vi "Convert Error Cluster to Table.vi"(11 "Error Codes":cluster{i32, string}[](array[cluster])) -> (2 "Code":i32[](array[numeric]), 3 "String":string[](array[string]))   [LabVIEW 2019, in "Protection and Counter Addon System Explorer.lvlib"] (continued)
(Hex 0xFFFFFCB6) The timed structure failed to unreserve the NI Scan Engine."}, {-841, "LabVIEW: (Hex 0xFFFFFCB7) The timed structure failed to retrieve the NI Scan Engine mode."}, {-840, "LabVIEW: (Hex 0xFFFFFCB8) The timed structure failed to reserve the NI Scan Engine."}, {-832, "LabVIEW: (Hex 0xFFFFFCC0) The Priority Mapper Table is full."}, {-831, "LabVIEW: (Hex 0xFFFFFCC1) Timing Source Fire Count Overflow"}, {-830, "LabVIEW: (Hex 0xFFFFFCC2) Invalid Trigger ID"}, {-826, "LabVIEW: (Hex 0xFFFFFCC6) A time-critical VI contains a timed structure."}, {-825, "LabVIEW: (Hex 0xFFFFFCC7) Invalid CPU Specified for timed structure."}, {-823, "LabVIEW: (Hex 0xFFFFFCC9) Cannot load Timed Loop Scheduler Dynamic Library."}, {-822, "LabVIEW: (Hex 0xFFFFFCCA) The timed structure feature or type is not supported on the current platform for the following timing source."}, {-821, "LabVIEW: (Hex 0xFFFFFCCB) The following timed structures timed out while waiting for the synchronization group to synchronize all timed structures in the group."}, {-820, "LabVIEW: (Hex 0xFFFFFCCC) The following timed structure has been initialized with illegal parameters."}, {-819, "LabVIEW: (Hex 0xFFFFFCCD) An illegal mode has been specified for the following given Timed Loop."}, {-818, "LabVIEW: (Hex 0xFFFFFCCE) An illegal period, priority, deadline, offset, or start has been specified for the following timed structure."}, {-817, "LabVIEW: (Hex 0xFFFFFCCF) Timing Source error or attempted to execute another iteration of a Timed Loop that was already aborted due to an error of the following timing source."}, {-816, "LabVIEW: (Hex 0xFFFFFCD0) Timed structure aborted or attempted to execute another iteration of the following aborted Timed Loop."}, {-815, "LabVIEW: (Hex 0xFFFFFCD1) Cannot add timing source to the following active timing source hierarchy."}, {-814, "LabVIEW: (Hex 0xFFFFFCD2) Cannot add timed structure to the active timed structure synchronization group."}, {-813, "LabVIEW: (Hex 0xFFFFFCD3) The following timing source can be assigned to only one timing source hierarchy at a time."}, {-812, "LabVIEW: (Hex 0xFFFFFCD4) The following timed structure can only be assigned to one timed structure synchronization group at a time."}, {-811, "LabVIEW: (Hex 0xFFFFFCD5) The given name is already being used by another timing source hierarchy:"}, {-810, "LabVIEW: (Hex 0xFFFFFCD6) The given name is already being used by another timed structure synchronization group:"}, {-809, "LabVIEW: (Hex 0xFFFFFCD7) The given name is already being used by the following timing source."}, {-808, "LabVIEW: (Hex 0xFFFFFCD8) The given name is already being used by the following timed structure."}, {-807, "LabVIEW: (Hex 0xFFFFFCD9) The following timing source hierarchy does not exist possibly because the timing source hierarchy has never been created, has been cleared, or an illegal action was attempted."}, {-806, "LabVIEW: (Hex 0xFFFFFCDA) The following synchronization group does not exist possibly because the synchronization group has never been created, has been cleared, or an illegal action was attempted."}, {-805, "LabVIEW: (Hex 0xFFFFFCDB) The following timing source does not exist. This error might occur because the timing source was never created, has been cleared, or an illegal action was attempted. Use the Create Timing Source VI to create a Timed Loop timing source."}, {-804, "LabVIEW: (Hex 0xFFFFFCDC) The timed structure does not exist, possibly because the timed structure has not been created, the timed structure has been cleared, or an illegal operation was attempted."}, {-803, "LabVIEW: (Hex 0xFFFFFCDD) Creating a new timing source hierarchy exceeds the maximum allowed number of simultaneously active timing source hierarchies."}, {-802, "LabVIEW: (Hex 0xFFFFFCDE) Creating another timed structure synchronization group exceeds the maximum allowed number of simultaneously active synchronization groups."}, {-801, "LabVIEW: (Hex 0xFFFFFCDF) Creating another timing source exceeds the maximum allowed number of simultaneously active timing sources."}, {-800, "LabVIEW: (Hex 0xFFFFFCE0) Creating another timed structure exceeds the maximum allowed number of simultaneously active timed structures."}, {-722, "LabVIEW: (Hex 0xFFFFFD2E) The TEDS bitstream is invalid or corrupt."}, {-721, "LabVIEW: (Hex 0xFFFFFD2F) The specified index is outside the bounds of the TEDS data array."}, {-720, "LabVIEW: (Hex 0xFFFFFD30) The specified value is outside of the acceptable range for this property."}, {-719, "LabVIEW: (Hex 0xFFFFFD31) The Basic TEDS was not found in the TEDS data."}, {-718, "LabVIEW: (Hex 0xFFFFFD32) LabVIEW is unable to locate the specified SelectCase or StructArray."}, {-717, "LabVIEW: (Hex 0xFFFFFD33) The specified VTEDS file was written with an incompatible version of the TEDS library."}, {-716, "LabVIEW: (Hex 0xFFFFFD34) The EEPROM is too small for data."}, {-715, "LabVIEW: (Hex 0xFFFFFD35) EEPROM Write Failure"}, {-714, "LabVIEW: (Hex 0xFFFFFD36) Bad EEPROM ID"}, {-713, "LabVIEW: (Hex 0xFFFFFD37) No EEPROM is detected."}, {-712, "LabVIEW: (Hex 0xFFFFFD38) This property cannot be edited because it is a constant in the template for this sensor."}, {-711, "LabVIEW: (Hex 0xFFFFFD39) The enumeration for this property does not correspond to the data type specified by the template."}, {-710, "LabVIEW: (Hex 0xFFFFFD3A) This TEDS sensor requires a manufacturer defined template."}, {-709, "LabVIEW: (Hex 0xFFFFFD3B) The specified property is a floating-point data type according to the template. Casting this property to an unsigned integer will result in a loss of precision."}, {-708, "LabVIEW: (Hex 0xFFFFFD3C) The specified property is specified by the TEDS template as a string data type and cannot be converted to a numeric."}, {-707, "LabVIEW: (Hex 0xFFFFFD3D) The TEDS user data does not contain 7-bit ASCII code."}, {-706, "LabVIEW: (Hex 0xFFFFFD3E) The requested property cannot be found in the current TEDS data."}, {-705, "LabVIEW: (Hex 0xFFFFFD3F) The template to decode the remainder of the TEDS bitstream cannot be found in the specified template directory."}, {-704, "LabVIEW: (Hex 0xFFFFFD40) The header selector in the legacy Basic TEDS is outside the acceptable range."}, {-703, "LabVIEW: (Hex 0xFFFFFD41) The TEDS data checksum is invalid."}, {-702, "LabVIEW: (Hex 0xFFFFFD42) This VI does not support the data type for this property."}, {-701, "LabVIEW: (Hex 0xFFFFFD43) The number of bits required for the requested action is not divisible by five."}, {-700, "LabVIEW: (Hex 0xFFFFFD44) The number of bits required is not divisible by seven."}, {-620, "LabVIEW: (Hex 0xFFFFFD94) Networked machine was not found."}, {-619, "LabVIEW: (Hex 0xFFFFFD95) Remote registry services not available or remote administration not enabled."}, {-618, "LabVIEW: (Hex 0xFFFFFD96) Cannot create a stable subkey under a volatile parent key."}, {-617, "LabVIEW: (Hex 0xFFFFFD97) Cannot create a symbolic link in a registry key that already has subkeys or values."}, {-616, "LabVIEW: (Hex 0xFFFFFD98) System could not allocate the required space in a registry log."}, {-615, "LabVIEW: (Hex 0xFFFFFD99) Illegal operation attempted on a registry key that has been marked for deletion."}, {-614, "LabVIEW: (Hex 0xFFFFFD9A) The system has attempted to load or restore a file into the registry, but the specified file is not in a registry file format."}, {-613, "LabVIEW: (Hex 0xFFFFFD9B) An I/O operation initiated by the registry failed irrecoverably. The registry could not read in, or write out, or flush, one of the files that contain the system's image of the registry."}, {-612, "LabVIEW: (Hex 0xFFFFFD9C) The registry is corrupted. The structure of one of the files that contains registry data is corrupted, the system's image of the file in memory is corrupted, or the file could not be recovered because the alternate copy or log was absent or corrupted."}, {-611, "LabVIEW: (Hex 0xFFFFFD9D) One of the files in the registry database had to be recovered by use of a log or alternate copy. The recovery was successful."}, {-610, "LabVIEW: (Hex 0xFFFFFD9E) The configuration registry key could not be written."}, {-609, "LabVIEW: (Hex 0xFFFFFD9F) The configuration registry key could not be read."}, {-608, "LabVIEW: (Hex 0xFFFFFDA0) The configuration registry key could not be opened."}, {-607, "LabVIEW: (Hex 0xFFFFFDA1) The configuration registry key is invalid."}, {-606, "LabVIEW: (Hex 0xFFFFFDA2) The configuration registry database is corrupt."}, {-605, "LabVIEW: (Hex 0xFFFFFDA3) Attempted to read beyond last key or value."}, {-604, "LabVIEW: (Hex 0xFFFFFDA4) Remote registry access denied."}, {-603, "LabVIEW: (Hex 0xFFFFFDA5) Specified key or value does not exist."}, {-602, "LabVIEW: (Hex 0xFFFFFDA6) Invalid registry refnum."}, {-601, "LabVIEW: (Hex 0xFFFFFDA7) Incorrect data type specified."}, {-600, "LabVIEW: (Hex 0xFFFFFDA8) Undetermined Windows registry error."}, {0, "LabVIEW: (Hex 0x0) Error connecting to GPIB driver or device. The NI-488.2 driver may not be installed."}, {1, "LabVIEW: (Hex 0x1) An input parameter is invalid. For example if the input is a path, the path might contain a character not allowed by the OS such as ? or @."}, {2, "LabVIEW: (Hex 0x2) Memory is full."}, {3, "LabVIEW: (Hex 0x3) Internal error. Wrong memory zone accessed."}, {4, "LabVIEW: (Hex 0x4) End of file encountered."}, {5, "LabVIEW: (Hex 0x5) File already open."}, {6, "LabVIEW: (Hex 0x6) Generic file I/O error."}, {7, "LabVIEW: (Hex 0x7) File not found. The file might be in a different location or deleted. Use the command prompt or the file explorer to verify that the path is correct."}, {8, "LabVIEW: (Hex 0x8) File permission error. You do not have the correct permissions for the file."}, {9, "LabVIEW: (Hex 0x9) Disk full. The disk or hard drive does not have enough free space to complete the operation. Try freeing up disk space or saving to a different disk or drive."}, {10, "LabVIEW: (Hex 0xA) Duplicate path."}, {11, "LabVIEW: (Hex 0xB) Too many files open."}, {12, "LabVIEW: (Hex 0xC) Some system capacity necessary for operation is not enabled."}, {13, "LabVIEW: (Hex 0xD) Failed to load dynamic library because of missing external symbols or dependencies, or because of an invalid file format."}, {14, "LabVIEW: (Hex 0xE) Cannot add resource."}, {15, "LabVIEW: (Hex 0xF) Resource not found."}, {16, "LabVIEW: (Hex 0x10) Image not found."}, {17, "LabVIEW: (Hex 0x11) Not enough memory to manipulate image."}, {18, "LabVIEW: (Hex 0x12) Pen does not exist."}, {19, "LabVIEW: (Hex 0x13) Configuration type invalid."}, {20, "LabVIEW: (Hex 0x14) Configuration token not found."}, {21, "LabVIEW: (Hex 0x15) Error occurred parsing configuration string."}, {22, "LabVIEW: (Hex 0x16) Configuration memory error."}, {23, "LabVIEW: (Hex 0x17) Bad external code format."}, {24, "LabVIEW: (Hex 0x18) External subroutine not supported."}, {25, "LabVIEW: (Hex 0x19) External code not present."}, {26, "LabVIEW: (Hex 0x1A) Null window."}, {27, "LabVIEW: (Hex 0x1B) Destroy window error."}, {28, "LabVIEW: (Hex 0x1C) Null menu."}, {29, "LabVIEW: (Hex 0x1D) Print aborted."}, {30, "LabVIEW: (Hex 0x1E) Bad print record."}, {31, "LabVIEW: (Hex 0x1F) Print driver error."}, {32, "LabVIEW: (Hex 0x20) Operating system error during print."}, {33, "LabVIEW: (Hex 0x21) Memory error during print."}, {34, "LabVIEW: (Hex 0x22) Print dialog error."}, {35, "LabVIEW: (Hex 0x23) Generic print error."}, {36, "LabVIEW: (Hex 0x24) Invalid device refnum."}, {37, "LabVIEW: (Hex 0x25) Device not found."}, {38, "LabVIEW: (Hex 0x26) Device parameter error."}, {39, "LabVIEW: (Hex 0x27) Device unit error."}, {40, "LabVIEW: (Hex 0x28) Cannot open device."}, {41, "LabVIEW: (Hex 0x29) Device call aborted."}, {42, "LabVIEW: (Hex 0x2A) Generic error."}, {43, "LabVIEW: (Hex 0x2B) Operation cancelled by user."}, {44, "LabVIEW: (Hex 0x2C) Object ID too low."}, {45, "LabVIEW: (Hex 0x2D) Object ID too high."}, {46, "LabVIEW: (Hex 0x2E) Object not in heap."}, {47, "LabVIEW: (Hex 0x2F) Unknown heap."}, {48, "LabVIEW: (Hex 0x30) Unknown object (invalid DefProc)."}, {49, "LabVIEW: (Hex 0x31) Unknown object (DefProc not in table)."}, {50, "LabVIEW: (Hex 0x32) Message out of range."}, {51, "LabVIEW: (Hex 0x33) Null method."}, {52, "LabVIEW: (Hex 0x34) Unknown message."}, {53, "LabVIEW: (Hex 0x35) Manager call not supported."}, {54, "LabVIEW: (Hex 0x36) The network address is ill-formed. Make sure the address is in a valid format. For TCP/IP, the address can be either a machine name or an IP address in the form xxx.xxx.xxx.xxx. If this error occurs when specifying a machine name, make sure the machine name is valid. Try to ping the machine name. Check that you have a DNS server properly configured. If you are using the TCP Open Connection function, ensure that the value of the remote port or service name is not 0."}, {55, "LabVIEW: (Hex 0x37) The network operation is in progress."}, {56, "LabVIEW: (Hex 0x38) The network operation exceeded the user-specified or system time limit."}, {57, "LabVIEW: (Hex 0x39) The network connection is busy."}, {58, "LabVIEW: (Hex 0x3A) The network function is not supported by the system."}, {59, "LabVIEW: (Hex 0x3B) The network is down, unreachable, or has been reset."}, {60, "LabVIEW: (Hex 0x3C) The specified port or network address is currently in use. Select an available port or network address."}, {61, "LabVIEW: (Hex 0x3D) Serial port parity error."}, {61, "LabVIEW: (Hex 0x3D) The system could not allocate the necessary memory."}, {62, "LabVIEW: (Hex 0x3E) Serial port overrun error."}, {62, "LabVIEW: (Hex 0x3E) The system caused the network connection to be aborted."}, {63, "LabVIEW: (Hex 0x3F) Serial port receive buffer overflow."}, {63, "LabVIEW: (Hex 0x3F) The network connection was refused by the server."}, {64, "LabVIEW: (Hex 0x40) Serial port framing error."}, {64, "LabVIEW: (Hex 0x40) The network connection is not yet established."}, {65, "LabVIEW: (Hex 0x41) Serial port timeout; bytes not received at serial port."}, {65, "LabVIEW: (Hex 0x41) The network connection is already established."}, {66, "LabVIEW: (Hex 0x42) The network connection was closed by the peer. If you are using the Open VI Reference function on a remote VI Server connection, verify that the machine is allowed access by selecting <b>Tools>>Options>>VI Server</b> on the server side."}, {67, "LabVIEW: (Hex 0x43) Interapplication Manager initialization error."}, {68, "LabVIEW: (Hex 0x44) Bad occurrence."}, {69, "LabVIEW: (Hex 0x45) Handler does not know what occurrence to wait for."}, {70, "LabVIEW: (Hex 0x46) Occurrence queue overflow."}, {71, "LabVIEW: (Hex 0x47) File datalog type conflict."}, {72, "LabVIEW: (Hex 0x48) Semaphore not signaled."}, {73, "LabVIEW: (Hex 0x49) Interapplication Manager unrecognized type error."}, {74, "LabVIEW: (Hex 0x4A) Memory or data structure corrupt."}, {75, "LabVIEW: (Hex 0x4B) Failed to make temporary DLL."}, {76, "LabVIEW: (Hex 0x4C) Old CIN version."}, {81, "LabVIEW: (Hex 0x51) Format specifier type mismatch."}, {82, "LabVIEW: (Hex 0x52) Unknown format specifier."}, {83, "LabVIEW: (Hex 0x53) Too few format specifiers."}, {84, "LabVIEW: (Hex 0x54) Too many format specifiers."}, {85, "LabVIEW: (Hex 0x55) Scan failed. The input string does not contain data in the expected format."}, {87, "LabVIEW: (Hex 0x57) Error converting to variant."}, {88, "LabVIEW: (Hex 0x58) Run-time menu error."}, {89, "LabVIEW: (Hex 0x59) Another user tampered with the VI password."}, {90, "LabVIEW: (Hex 0x5A) Variant attribute not found."}, {91, "LabVIEW: (Hex 0x5B) The data type of the variant is not compatible with the data type wired to the type input."}, {92, "LabVIEW: (Hex 0x5C) The ActiveX event data was not available on the queue."}, {93, "LabVIEW: (Hex 0x5D) ActiveX event information was not available."}, {94, "LabVIEW: (Hex 0x5E) The occurrence associated with the ActiveX event was not found."}, {95, "LabVIEW: (Hex 0x5F) The ActiveX event queue could not be created."}, {96, "LabVIEW: (Hex 0x60) ActiveX event information was not available in the type library."}, {97, "LabVIEW: (Hex 0x61) A null or previously deleted refnum was passed in as an input."}, {98, "LabVIEW: (Hex 0x62) Incorrect file type. Attempted to read from or write to a file of a type incompatible with the operation. This normally is a user data file."}, {99, "LabVIEW: (Hex 0x63) Incorrect file version. Attempted to read from or write to a file of a version incompatible with the write/read function version. This file normally is a user data file."}, {100, "LabVIEW: (Hex 0x64) File contains erroneous data. This normally is a user data file."}, {102, "LabVIEW: (Hex 0x66) IVI invalid downcast."}, {103, "LabVIEW: (Hex 0x67) No IVI class session opened.  You must call the class driver Initialize VI before you can call a specific driver VI.  This error also can occur if the IVI Logical Name control is set to the wrong IVI Class."}, {108, "LabVIEW: (Hex 0x6C) Singlecast connections cannot send to multicast addresses."}, {109, "LabVIEW: (Hex 0x6D) Multicast connections cannot send to singlecast addresses."}, {110, "LabVIEW: (Hex 0x6E) Specified IP address is not in multicast address range."}, {111, "LabVIEW: (Hex 0x6F) Cannot write to read-only multicast connection."}, {112, "LabVIEW: (Hex 0x70) Cannot read from write-only multicast connection."}, {113, "LabVIEW: (Hex 0x71) A message sent on a datagram socket was larger than the internal message buffer or some other network limit, or the buffer used to receive a datagram was smaller than the datagram itself."}, {114, "LabVIEW: (Hex 0x72) Could not create TCP listener port because the port, service name, or net address conflict with a TCP listener that already exists."}, {116, "LabVIEW: (Hex 0x74) Unflatten or byte stream read operation failed due to corrupt, unexpected, or truncated data."}, {117, "LabVIEW: (Hex 0x75) Directory path supplied where a file path is required."}, {118, "LabVIEW: (Hex 0x76) The supplied folder path does not exist."}, {119, "LabVIEW: (Hex 0x77) Illegal combination of Bluetooth discoverable and non-connectable modes."}, {120, "LabVIEW: (Hex 0x78) Error setting Bluetooth mode."}, {121, "LabVIEW: (Hex 0x79) Invalid GUID string."}, {122, "LabVIEW: (Hex 0x7A) The resource you are attempting to open was created in a more recent version of LabVIEW and is incompatible with this version."}, {123, "LabVIEW: (Hex 0x7B) A timeout occurred."}, {124, "LabVIEW: (Hex 0x7C) A string contained an unexpected null character."}, {125, "LabVIEW: (Hex 0x7D) A stack overflow occurred."}, {126, "LabVIEW: (Hex 0x7E) Could not query socket state."}, {127, "LabVIEW: (Hex 0x7F) The specified socket is not an IPv4 socket."}, {128, "LabVIEW: (Hex 0x80) Open connection limit exceeded."}, {129, "LabVIEW: (Hex 0x81) The path to access is too long for the current operating system."}, {130, "LabVIEW: (Hex 0x82) Operation attempted to create a set with duplicate elements. All elements of a set must be unique."}, {131, "LabVIEW: (Hex 0x83) Operation attempted to create a map with duplicate keys. All keys of a map must be unique."}, {824, "LabVIEW: (Hex 0x338) You must  supply a mode to change the offset of the Timed Loop."}, {1000, "LabVIEW: (Hex 0x3E8) The VI is not in a state compatible with this operation."}, {1001, "LabVIEW: (Hex 0x3E9) The VI front panel is not open."}, {1002, "LabVIEW: (Hex 0x3EA) The VI cannot run because it has a front panel control in an error state."}, {1003, "LabVIEW: (Hex 0x3EB) The VI is not executable.  This error may occur because the VI is either broken or contains a subVI that LabVIEW cannot locate. Select <b>File>>Open</b> to open the VI and verify that you can run it."}, {1004, "LabVIEW: (Hex 0x3EC) The VI is not in memory."}, {1005, "LabVIEW: (Hex 0x3ED) VI execution has been disabled in the <b>VI Properties</b> dialog box."}, {1006, "LabVIEW: (Hex 0x3EE) FPDCO on connector pane thinks it is constant."}, {1007, "LabVIEW: (Hex 0x3EF) No IP record in summary."}, {1008, "LabVIEW: (Hex 0x3F0) Cannot load connector pane."}, {1009, "LabVIEW: (Hex 0x3F1) Variant tag out of range."}, {1010, "LabVIEW: (Hex 0x3F2) No default or operate data."}, {1011, "LabVIEW: (Hex 0x3F3) VI Creation failed."}, {1012, "LabVIEW: (Hex 0x3F4) Cannot load block diagram."}, {1013, "LabVIEW: (Hex 0x3F5) Cannot load front panel."}, {1014, "LabVIEW: (Hex 0x3F6) Linker error."}, {1015, "LabVIEW: (Hex 0x3F7) Printer is not responding. Check printer configuration."}, {1016, "LabVIEW: (Hex 0x3F8) Cannot load History."}, {1017, "LabVIEW: (Hex 0x3F9) VI has been modified on disk since it was last loaded or saved."}, {1018, "LabVIEW: (Hex 0x3FA) Unspecified error occurred."}, {1019, "LabVIEW: (Hex 0x3FB) One or more untitled subVIs exist. This file cannot be saved until all dependent files have been named."}, {1020, "LabVIEW: (Hex 0x3FC) This CIN can only be invoked from a registered wizard."}, {1021, "LabVIEW: (Hex 0x3FD) Illegal Object Id passed to wizard CIN."}, {1022, "LabVIEW: (Hex 0x3FE) Wizard Template not found."}, {1023, "LabVIEW: (Hex 0x3FF) Wizard template does not have a diagram."}, {1024, "LabVIEW: (Hex 0x400) Call Instrument aborted."}, {1025, "LabVIEW: (Hex 0x401) Application Reference is invalid."}, {1026, "LabVIEW: (Hex 0x402) VI Reference is invalid."}, {1027, "LabVIEW: (Hex 0x403) For the requested operation, the reference cannot be reserved as requested, is in an improper reservation mode, or the execution state must be set to running or reserved."}, {1028, "LabVIEW: (Hex 0x404) Attribute selector is invalid."}, {1029, "LabVIEW: (Hex 0x405) VI Server property is read-only."}, {1030, "LabVIEW: (Hex 0x406) VI Reference is already reserved for editing."}, {1031, "LabVIEW: (Hex 0x407) VI Reference type does not match VI connector pane."}, {1032, "LabVIEW: (Hex 0x408) VI Server access denied."}, {1033, "LabVIEW: (Hex 0x409) Bad run-time menu file version."}, {1034, "LabVIEW: (Hex 0x40A) Bad run-time menu file."}, {1035, "LabVIEW: (Hex 0x40B) Operation is invalid for this type of VI."}, {1036, "LabVIEW: (Hex 0x40C) Method selector is invalid."}, {1037, "LabVIEW: (Hex 0x40D) Incompatible VI Server protocol version."}, {1038, "LabVIEW: (Hex 0x40E) Required parameter missing."}, {1039, "LabVIEW: (Hex 0x40F) VI was aborted."}, {1040, "LabVIEW: (Hex 0x410) VI is password protected."}, {1041, "LabVIEW: (Hex 0x411) Incorrect password."}, {1042, "LabVIEW: (Hex 0x412) Attempted recursive call."}, {1043, "LabVIEW: (Hex 0x413) The property or method is not supported in this version of LabVIEW."}, {1044, "LabVIEW: (Hex 0x414) VI is locked."}, {1045, "LabVIEW: (Hex 0x415) Null Refnum passed to Close Reference."}, {1046, "LabVIEW: (Hex 0x416) LabVIEW cannot initialize the script server.  Ensure the server software is installed."}, {1047, "LabVIEW: (Hex 0x417) LabVIEW failed to send variable to the script server."}, {1048, "LabVIEW: (Hex 0x418) LabVIEW failed to get variable from the script server."}, {1049, "LabVIEW: (Hex 0x419) LabVIEW failed to send script text to the script server."}, {1050, "LabVIEW: (Hex 0x41A) Error occurred while executing script."}, {1051, "LabVIEW: (Hex 0x41B) A LabVIEW file of that name already exists in memory, or exists within a project library already in memory."}, {1052, "LabVIEW: (Hex 0x41C) The LabVIEW filename is invalid."}, {1053, "LabVIEW: (Hex 0x41D) At run time, LabVIEW cannot find script support DLL."}, {1054, "LabVIEW: (Hex 0x41E) The specified object was not found."}, {1055, "LabVIEW: (Hex 0x41F) Object reference is invalid."}, {1056, "LabVIEW: (Hex 0x420) Specified object is not scriptable in this version."}, {1057, "LabVIEW: (Hex 0x421) Type mismatch: Object cannot be cast to the specified type."}, {1058, "LabVIEW: (Hex 0x422) Specified property not found."}, {1059, "LabVIEW: (Hex 0x423) Unexpected file type."}, {1060, "LabVIEW: (Hex 0x424) Object cannot contain (own) the specified object."}, {1061, "LabVIEW: (Hex 0x425) Unable to create new object."}, {1062, "LabVIEW: (Hex 0x426) Specified objects cannot be wired together."}, {1063, "LabVIEW: (Hex 0x427) Specified terminal not found in the object."}, {1064, "LabVIEW: (Hex 0x428) The specified VI may not be saved for previous because it resides in the vi.lib directory."}, {1065, "LabVIEW: (Hex 0x429) The path to the VI to save is an empty or relative path.  It must be an absolute path."}, {1066, "LabVIEW: (Hex 0x42A) Hardware open error."}, {1067, "LabVIEW: (Hex 0x42B) Hardware close error."}, {1068, "LabVIEW: (Hex 0x42C) Hardware transact error."}, {1069, "LabVIEW: (Hex 0x42D) Hardware DLL missing."}, {1070, "LabVIEW: (Hex 0x42E) Hardware no session error."}, {1071, "LabVIEW: (Hex 0x42F) LabVIEW cannot locate the specified method."}, {1072, "LabVIEW: (Hex 0x430) This property or method is not yet implemented."}, {1073, "LabVIEW: (Hex 0x431) This property is writable only when the VI is in edit mode, or this method is available only when the VI is in edit mode."}, {1074, "LabVIEW: (Hex 0x432) Cannot create a control/indicator for the specified terminal."}, {1075, "LabVIEW: (Hex 0x433) Cannot create a constant for the specified terminal."}, {1076, "LabVIEW: (Hex 0x434) VI is not debuggable."}, {1077, "LabVIEW: (Hex 0x435) Invalid property value."}, {1078, "LabVIEW: (Hex 0x436) Failed to load shared library %s. Ensure that the library is present on the RT target. Use either MAX to install NI software or FTP to transfer custom libraries to the RT target."}, {1079, "LabVIEW: (Hex 0x437) When the RT target booted, the startup application configured to launch was missing."}, {1080, "LabVIEW: (Hex 0x438) The startup application configured to launch was corrupt and failed to load when the RT target booted."}, {1081, "LabVIEW: (Hex 0x439) Exception caused by loading of library %s on RT target device."}, {1082, "LabVIEW: (Hex 0x43A) Operation not valid for strict type definition instance."}, {1083, "LabVIEW: (Hex 0x43B) Invalid connector pane pattern."}, {1084, "LabVIEW: (Hex 0x43C) Specified control or indicator cannot be hooked up to the connector pane."}, {1085, "LabVIEW: (Hex 0x43D) Invalid connector terminal."}, {1086, "LabVIEW: (Hex 0x43E) Wrong control type."}, {1087, "LabVIEW: (Hex 0x43F) There is no DataSocket information available for the object."}, {1088, "LabVIEW: (Hex 0x440) Bad value for parameter."}, {1089, "LabVIEW: (Hex 0x441) Error occurred while executing script. Error message from server: %s."}, {1090, "LabVIEW: (Hex 0x442) Specified object cannot be moved."}, {1091, "LabVIEW: (Hex 0x443) The VI Server or client received an unrecognized message."}, {1092, "LabVIEW: (Hex 0x444) Invalid Class Operator VI."}, {1093, "LabVIEW: (Hex 0x445) Specified object is not deletable."}, {1094, "LabVIEW: (Hex 0x446) Queue and notifier references of the same name must be obtained using the same data type."}, {1095, "LabVIEW: (Hex 0x447) This container cannot be left without a subtype. Right-click the container border and select Replace or drag new subtype."}, {1096, "LabVIEW: (Hex 0x448) The Open VI Reference function cannot prepare a non-reentrant VI for reentrant run."}, {1097, "LabVIEW: (Hex 0x449) An exception occurred within the external code called by a Call Library Function Node. The exception might have corrupted the LabVIEW memory. Save any work to a new location and restart LabVIEW."}, {1098, "LabVIEW: (Hex 0x44A) Cannot disconnect type definitions or polymorphic VIs if the block diagram is not available."}, {1099, "LabVIEW: (Hex 0x44B) Scripting: SubVI is not loaded."}, {1100, "LabVIEW: (Hex 0x44C) No object of that name was found. No reference could be returned."}, {1101, "LabVIEW: (Hex 0x44D) Insufficient privileges to read, write, or create an item in the DataSocket Server. Use the DataSocket Server Manager to configure these privileges."}, {1102, "LabVIEW: (Hex 0x44E) The string wired to the <b>xml string</b> input is empty."}, {1103, "LabVIEW: (Hex 0x44F) The XML tag describing the type of data is not recognized."}, {1104, "LabVIEW: (Hex 0x450) No end tag was found for an XML start/end tag pair."}, {1105, "LabVIEW: (Hex 0x451) An unknown or unexpected XML tag was discovered."}, {1106, "LabVIEW: (Hex 0x452) The XML tag describing the type of data does not match the wired type."}, {1107, "LabVIEW: (Hex 0x453) The XML enumerated type choice(s) does not match the wired type."}, {1108, "LabVIEW: (Hex 0x454) XML value text is illegal or out of range for type and/or format."}, {1109, "LabVIEW: (Hex 0x455) Unsupported data type."}, {1110, "LabVIEW: (Hex 0x456) No longer used."}, {1111, "LabVIEW: (Hex 0x457) Release Semaphore called on a semaphore that was not currently acquired."}, {1112, "LabVIEW: (Hex 0x458) Internal Error. No class manager found for the type requested."}, {1113, "LabVIEW: (Hex 0x459) Internal Error. The external object class was not found."}, {1114, "LabVIEW: (Hex 0x45A) This item is read-only. You must connect in read mode."}, {1115, "LabVIEW: (Hex 0x45B) This item is write-only. You must connect in write mode."}, {1116, "LabVIEW: (Hex 0x45C) RTTarget.DiskCache.SizeInKB config token must be greater than zero."}, {1117, "LabVIEW: (Hex 0x45D) RTTarget.DiskCache.Thread.Priority config token must be between -2 and 2."}, {1118, "LabVIEW: (Hex 0x45E) RTTarget.DiskCache.Thread.IntervalInSecs config token must be greater than zero."}, {1119, "LabVIEW: (Hex 0x45F) RTTarget.DiskCache.Thread.LinePerWakeup config token must be greater than or equal to zero."}, {1120, "LabVIEW: (Hex 0x460) Not enough memory to create disk cache."}, {1121, "LabVIEW: (Hex 0x461) Cannot create disk cache flush thread."}, {1122, "LabVIEW: (Hex 0x462) Refnum became invalid while node waited for it."}, {1123, "LabVIEW: (Hex 0x463) You cannot create an object (such as control caption) in built applications. You must create these objects in the LabVIEW development system."}, {1124, "LabVIEW: (Hex 0x464) VI is not loadable.\n\nIn a built application, this error might occur because the VI being loaded was last compiled for a different OS or with CPU features, such as SSE, that this target does not support. In this case you must rebuild the application for the target OS and make sure SSE compiler settings in the build specifications match the target platform. This error also might occur if the VI is a polymorphic VI, which cannot be loaded in the LabVIEW Run-Time Engine. You must load an instance of the polymorphic VI instead of the polymorphic VI itself."}, {1125, "LabVIEW: (Hex 0x465) File version is later than the current LabVIEW version."}, {1126, "LabVIEW: (Hex 0x466) VI version is too early to convert to the current LabVIEW version."}, {1127, "LabVIEW: (Hex 0x467) Cannot instantiate template VI because it is already in memory."}, {1128, "LabVIEW: (Hex 0x468) Input unit is not compatible with the current unit."}, {1129, "LabVIEW: (Hex 0x469) You cannot assign the same numeric value to two or more strings in a ring control. You also cannot assign the same string value to two or more strings in a combo box control."}, {1130, "LabVIEW: (Hex 0x46A) The VI Server connection peer is unresponsive. Refer to the Connection Responsiveness: Check Method topic in the LabVIEW Help for more information about connection polling."}, {1131, "LabVIEW: (Hex 0x46B) You cannot use this property with this system control."}, {1132, "LabVIEW: (Hex 0x46C) Busy with another operation."}, {1133, "LabVIEW: (Hex 0x46D) LabVIEW is busy connecting."}, {1134, "LabVIEW: (Hex 0x46E) A different read operation is in progress."}, {1135, "LabVIEW: (Hex 0x46F) The tree control's active item is not valid for this property."}, {1136, "LabVIEW: (Hex 0x470) You wired an invalid item tag to a tree control property or method."}, {1137, "LabVIEW: (Hex 0x471) Tree control's internal data is corrupt."}, {1138, "LabVIEW: (Hex 0x472) An exception occurred within external code called by LabVIEW. This might have corrupted the LabVIEW memory. Save any work to a new location and restart LabVIEW."}, {1139, "LabVIEW: (Hex 0x473) A DataSocket item name cannot contain certain characters."}, {1140, "LabVIEW: (Hex 0x474) Exceeded maximum DataSocket item count. Use the DataSocket Server Manager to change the maximum number of dynamically created items the data server will allow."}, {1141, "LabVIEW: (Hex 0x475) Exceeded maximum data item connection count. Use the DataSocket Server Manager to change the maximum number of connections the data server will allow."}, {1142, "LabVIEW: (Hex 0x476) Multiple writers are not allowed."}, {1143, "LabVIEW: (Hex 0x477) Cannot load dataskt.llb."}, {1144, "LabVIEW: (Hex 0x478) Cannot insert VI in a subpanel control because VI is already open."}, {1145, "LabVIEW: (Hex 0x479) Cannot open VI because it is already in a subpanel control."}, {1146, "LabVIEW: (Hex 0x47A) You attempted an operation that would change a child-only item into a parent item."}, {1147, "LabVIEW: (Hex 0x47B) Cannot insert a remote VI in a subpanel control."}, {1148, "LabVIEW: (Hex 0x47C) This property is read only while the VI is in a subpanel."}, {1149, "LabVIEW: (Hex 0x47D) Cannot close or set the state of a closed front panel. The front panel must already be open before you close it or set its state."}, {1150, "LabVIEW: (Hex 0x47E) Cannot open a front panel that is already open. To set the state of the open front panel, use the Front Panel Window:State property."}, {1151, "LabVIEW: (Hex 0x47F) Invalid input for front panel state."}, {1152, "LabVIEW: (Hex 0x480) Cannot replace a locked object."}, {1153, "LabVIEW: (Hex 0x481) Cannot replace object inside a group."}, {1154, "LabVIEW: (Hex 0x482) Cannot replace this object with the type specified."}, {1155, "LabVIEW: (Hex 0x483) Cannot insert the object of specified type into the wire."}, {1156, "LabVIEW: (Hex 0x484) Memory full error, possibly due to a data format not matching expected data type."}, {1157, "LabVIEW: (Hex 0x485) You cannot use this property with a numeric indicator."}, {1158, "LabVIEW: (Hex 0x486) One or more application items already exist."}, {1159, "LabVIEW: (Hex 0x487) Cannot find one or more application items."}, {1160, "LabVIEW: (Hex 0x488) Illegal menu."}, {1161, "LabVIEW: (Hex 0x489) Cannot find the menu because the front panel is not open."}, {1162, "LabVIEW: (Hex 0x48A) Cannot find one or more tags."}, {1163, "LabVIEW: (Hex 0x48B) Illegal shortcut."}, {1164, "LabVIEW: (Hex 0x48C) Cannot modify an application menu item."}, {1165, "LabVIEW: (Hex 0x48D) Cannot find the menu."}, {1166, "LabVIEW: (Hex 0x48E) One or more illegal menu item indexes."}, {1167, "LabVIEW: (Hex 0x48F) Cannot insert a group item as a menu bar item."}, {1168, "LabVIEW: (Hex 0x490) Exceeded the maximum number of menus for this platform. The VI will use the default run-time menu."}, {1169, "LabVIEW: (Hex 0x491) Cannot select the menu item because it is disabled or has a submenu attached to it."}, {1170, "LabVIEW: (Hex 0x492) INTERNAL TO LABVIEW ONLY. DO NOT DOCUMENT TO USERS. Used by Queues and Notifiers to signal a condition in which they do not need to wait on data."}, {1171, "LabVIEW: (Hex 0x493) You are attempting to start a new transaction when a transaction is currently underway. Please finish the current transaction before starting a new one."}, {1172, "LabVIEW: (Hex 0x494) A .NET exception occurred in an external assembly. For information about correcting this error, copy the following exception (in bold), and search the Microsoft Developer Network (MSDN) Web site or the Web for a possible explanation."}, {1173, "LabVIEW: (Hex 0x495) LabVIEW data type does not match the .NET type."}, {1174, "LabVIEW: (Hex 0x496) Invalid return parameter for Call Library Function Node. The return type must be Void, Numeric, or String. Numeric return types are passed by value. Strings return types are passed as a C String Pointer or a Pascal String Pointer."}, {1175, "LabVIEW: (Hex 0x497) Invalid array dimension in Call Library Function Node configuration. An array must have 1 or more dimensions."}, {1176, "LabVIEW: (Hex 0x498) Invalid waveform dimension in Call Library Function Node configuration. A waveform must have 0 or 1 dimensions."}, {1177, "LabVIEW: (Hex 0x499) Invalid data type for Call Library Function Node parameter. Void can be used only as return type of function."}, {1178, "LabVIEW: (Hex 0x49A) LabVIEW reached end of file."}, {1179, "LabVIEW: (Hex 0x49B) Access mode not supported for operation."}, {1180, "LabVIEW: (Hex 0x49C) Pending operation in progress."}, {1181, "LabVIEW: (Hex 0x49D) Protocol not recognized by LabVIEW."}, {1182, "LabVIEW: (Hex 0x49E) Error parsing URL."}, {1183, "LabVIEW: (Hex 0x49F) Synchronous operation not supported for connection.  Append \"?sync=true\" to URL to enable synchronous operations with the PSP protocol.  LabVIEW 8.0.1 and later support synchronous operations."}, {1184, "LabVIEW: (Hex 0x4A0) Path not found, FTP login incorrect, or no FTP write permission."}, {1185, "LabVIEW: (Hex 0x4A1) OPC item not found."}, {1186, "LabVIEW: (Hex 0x4A2) Cannot show or hide the label on its own. Label visibility is controlled by the label owner."}, {1187, "LabVIEW: (Hex 0x4A3) Internet Explorer is required for this operation but it is not installed."}, {1188, "LabVIEW: (Hex 0x4A4) The static VI reference is not configured."}, {1189, "LabVIEW: (Hex 0x4A5) You cannot register the same event on an object multiple times."}, {1190, "LabVIEW: (Hex 0x4A6) The operation is not allowed when the control has key focus."}, {1191, "LabVIEW: (Hex 0x4A7) The wire already has a probe on it."}, {1192, "LabVIEW: (Hex 0x4A8) No data range set for digital displays."}, {1193, "LabVIEW: (Hex 0x4A9) When a Boolean control has a latch mechanical action, you cannot use the Value property to read or write its value."}, {1194, "LabVIEW: (Hex 0x4AA) This Express VI requires DIAdem 8.1 or later and the LabVIEW DIAdem Connectivity VIs version 2.1 or later. The Connectivity VIs are available for free download from ni.com."}, {1195, "LabVIEW: (Hex 0x4AB) You must install the .NET Framework 4.0 for this operation."}, {1196, "LabVIEW: (Hex 0x4AC) Cannot list the same terminal more than once in the grown region of the expandable subVI."}, {1197, "LabVIEW: (Hex 0x4AD) This operation is not valid for static VI references. To run a VI using a static VI reference, use an Invoke Node to call the Run VI method."}, {1198, "LabVIEW: (Hex 0x4AE) The VI is not in a state compatible with this operation. Change the execution mode of the referenced VI to reentrant for this operation."}, {1199, "LabVIEW: (Hex 0x4AF) Cannot convert the specified LabVIEW type to  .NET object."}, {1301, "LabVIEW: (Hex 0x515) The dimension of the array passed in does not match the expected dimension for the operation."}, {1302, "LabVIEW: (Hex 0x516) The size of the array passed in does not match the expected size of the array for the operation."}, {1303, "LabVIEW: (Hex 0x517) The elements of the array are not unique. There are duplicated items in the array."}, {1304, "LabVIEW: (Hex 0x518) The array index is outside of the array bounds."}, {1305, "LabVIEW: (Hex 0x519) The required page cannot be found."}, {1306, "LabVIEW: (Hex 0x51A) Unable to load new code resource to the node. Code resource already loaded."}, {1307, "LabVIEW: (Hex 0x51B) Subpanel control could not open the VI window."}, {1308, "LabVIEW: (Hex 0x51C) The Property or Invoke Node is not linked to a front panel control."}, {1309, "LabVIEW: (Hex 0x51D) The Property or Invoke Node reference input terminal is already wired."}, {1310, "LabVIEW: (Hex 0x51E) The object is not in the same VI as the Property or Invoke Node."}, {1311, "LabVIEW: (Hex 0x51F) The input for class name is not correct or is in the wrong format."}, {1312, "LabVIEW: (Hex 0x520) Structure frame index is out of range."}, {1313, "LabVIEW: (Hex 0x521) You cannot use this property on a control in a radio buttons control."}, {1314, "LabVIEW: (Hex 0x522) You cannot use this property on an instance of a type definition set to update automatically from the master copy of the type definition."}, {1315, "LabVIEW: (Hex 0x523) You have attempted to create a data type with a descriptor that is too large."}, {1316, "LabVIEW: (Hex 0x524) Specified method not found."}, {1317, "LabVIEW: (Hex 0x525) LabVIEW cannot load the Facade VI."}, {1318, "LabVIEW: (Hex 0x526) Run-time menu shortcuts are not supported for this type of menu."}, {1319, "LabVIEW: (Hex 0x527) Cannot insert a VI into a subpanel that is not in a running state."}, {1320, "LabVIEW: (Hex 0x528) In run mode, LabVIEW cannot get or set a property for a control part that has not been created."}, {1321, "LabVIEW: (Hex 0x529) NI License Manager is not initialized."}, {1322, "LabVIEW: (Hex 0x52A) Invalid project build reference."}, {1323, "LabVIEW: (Hex 0x52B) Invalid project source item reference."}, {1324, "LabVIEW: (Hex 0x52C) The specified key is invalid."}, {1325, "LabVIEW: (Hex 0x52D) LabVIEW cannot find the specified event."}, {1326, "LabVIEW: (Hex 0x52E) The specified project item is invalid."}, {1327, "LabVIEW: (Hex 0x52F) The specified NIIM is invalid for the current project."}, {1328, "LabVIEW: (Hex 0x530) The instance of MAX associated with the project is invalid."}, {1329, "LabVIEW: (Hex 0x531) The server site associated with the project is invalid."}, {1330, "LabVIEW: (Hex 0x532) A provider associated with the project is invalid."}, {1331, "LabVIEW: (Hex 0x533) A service provider associated with the project is invalid."}, {1332, "LabVIEW: (Hex 0x534) The project site associated with the project is invalid."}, {1333, "LabVIEW: (Hex 0x535) The project reference does not refer to a valid project."}, {1334, "LabVIEW: (Hex 0x536) Unable to bind to the specified project item."}, {1335, "LabVIEW: (Hex 0x537) Unable to update the specified item UI."}, {1336, "LabVIEW: (Hex 0x538) The specified property is invalid."}, {1337, "LabVIEW: (Hex 0x539) Not enough memory to complete this remote panel operation."}, {1338, "LabVIEW: (Hex 0x53A) Network type not supported by remote panel protocol."}, {1339, "LabVIEW: (Hex 0x53B) Remote panel connection is closed."}, {1340, "LabVIEW: (Hex 0x53C) Invalid server IP address."}, {1341, "LabVIEW: (Hex 0x53D) Remote panel connection refused by the specified server."}, {1343, "LabVIEW: (Hex 0x53F) Client does not have access to remote panel server."}, {1344, "LabVIEW: (Hex 0x540) The remote panel protocol version is incompatible."}, {1345, "LabVIEW: (Hex 0x541) The LabVIEW client version is incompatible with the LabVIEW server version."}, {1346, "LabVIEW: (Hex 0x542) Server does not support remote panels."}, {1347, "LabVIEW: (Hex 0x543) You cannot connect to the local LabVIEW application."}, {1348, "LabVIEW: (Hex 0x544) Remote panel server failed to send the requested VI."}, {1349, "LabVIEW: (Hex 0x545) Client does not have access to specified VI."}, {1350, "LabVIEW: (Hex 0x546) Requested VI is broken and cannot be viewed or controlled."}, {1351, "LabVIEW: (Hex 0x547) Requested VI is not a standard VI. You cannot view or control a  polymorphic VI, custom control, or global variable VI remotely."}, {1352, "LabVIEW: (Hex 0x548) Requested VI is not loaded into memory on the server computer."}, {1353, "LabVIEW: (Hex 0x549) Requested VI is not in run mode."}, {1354, "LabVIEW: (Hex 0x54A) VI name required."}, {1355, "LabVIEW: (Hex 0x54B) Fatal error occurred during operation, closing connection."}, {1356, "LabVIEW: (Hex 0x54C) A remote panel connection does not exist for the specified VI."}, {1357, "LabVIEW: (Hex 0x54D) A LabVIEW file from that path already exists in memory, or exists within a project library already in memory."}, {1358, "LabVIEW: (Hex 0x54E) The splitter bar cannot be moved to this position because it violates the minimum or maximum size of a descendant pane."}, {1359, "LabVIEW: (Hex 0x54F) A drag cannot start because a previous drag transaction is still pending."}, {1360, "LabVIEW: (Hex 0x550) Cannot provide the type of data requested for this drag and drop operation."}, {1361, "LabVIEW: (Hex 0x551) The name or data type of a drag data element conflicts with the built-in LabVIEW drag data types."}, {1362, "LabVIEW: (Hex 0x552) Cannot use this property with this string display mode or if word wrapping is enabled."}, {1363, "LabVIEW: (Hex 0x553) The specified name or GUID is invalid."}, {1364, "LabVIEW: (Hex 0x554) The provider plug-in is not installed or somehow corrupt."}, {1365, "LabVIEW: (Hex 0x555) Failed to generate a valid GUID."}, {1366, "LabVIEW: (Hex 0x556) You cannot hide or show the scroll bars of a subpanel control when a VI containing multiple panels is inserted."}, {1367, "LabVIEW: (Hex 0x557) Unable to authenticate because the NI Security library failed to load."}, {1368, "LabVIEW: (Hex 0x558) Unable to authenticate because LabVIEW failed to load an NI Security library that is required to authenticate access."}, {1369, "LabVIEW: (Hex 0x559) Removing data connection from this control."}, {1370, "LabVIEW: (Hex 0x55A) The selected build failed to complete."}, {1371, "LabVIEW: (Hex 0x55B) Class library could not be loaded."}, {1372, "LabVIEW: (Hex 0x55C) Class private data control could not be loaded."}, {1373, "LabVIEW: (Hex 0x55D) Class could not be loaded."}, {1374, "LabVIEW: (Hex 0x55E) ScriptingLanguageError"}, {1375, "LabVIEW: (Hex 0x55F) The .NET Framework 4.0 is not  installed on this machine."}, {1376, "LabVIEW: (Hex 0x560) A Diagram Disable structure cannot have a default frame."}, {1377, "LabVIEW: (Hex 0x561) A Diagram Disable structure cannot have conditions."}, {1378, "LabVIEW: (Hex 0x562) Cannot set the Active Frame property on a Conditional Disable structure."}, {1379, "LabVIEW: (Hex 0x563) The user failed a security authentication check."}, {1380, "LabVIEW: (Hex 0x564) License checkout failure.  Unable to checkout the requested license feature because the license is invalid or does not exist."}, {1381, "LabVIEW: (Hex 0x565) Cannot create semaphores with a size less than one."}, {1382, "LabVIEW: (Hex 0x566) The Start Drag method failed because the control is configured to not allow dragging."}, {1383, "LabVIEW: (Hex 0x567) The data type of the data read does not match the data type of the type input."}, {1384, "LabVIEW: (Hex 0x568) Cannot start dragging because duplicate names for drag data types were passed to the Start Drag method or Drag Starting? event."}, {1385, "LabVIEW: (Hex 0x569) Cannot start a drag and drop operation because the data provided is invalid."}, {1386, "LabVIEW: (Hex 0x56A) The specified .NET class is not available in LabVIEW."}, {1387, "LabVIEW: (Hex 0x56B) The specified .NET assembly is not available in LabVIEW."}, {1388, "LabVIEW: (Hex 0x56C) The block diagram you are attempting to access belongs to a VI that is either in evaluation mode or has an invalid license."}, {1389, "LabVIEW: (Hex 0x56D) You are attempting to save or copy a VI that is either in evaluation mode or has an invalid license."}, {1390, "LabVIEW: (Hex 0x56E) You attempted to open a VI Server reference to an out-of-scope VI. A VI can open VI Server references only to other VIs that it could call as subVIs. After the reference is opened, that VI can return the reference to other VIs that could not normally open the reference."}, {1391, "LabVIEW: (Hex 0x56F) You cannot set a breakpoint on a Conditional Disable structure that resides on a simulation diagram."}, {1392, "LabVIEW: (Hex 0x570) LabVIEW classes do not support Revert if the library version has been bumped. There is insufficient information to undo a change to the live data in controls and indicators. To revert current changes, you must unload the class and all VIs that reference the class without saving any changes and then reload from disk."}, {1393, "LabVIEW: (Hex 0x571) The LabVIEW class is not in memory. This dynamic subVI cannot execute."}, {1394, "LabVIEW: (Hex 0x572) This dynamic subVI cannot execute because the needed member VI cannot be found."}, {1395, "LabVIEW: (Hex 0x573) The opening angle bracket was found in the open tag, but the closing angle bracket is missing from the open tag."}, {1396, "LabVIEW: (Hex 0x574) Cannot convert text from the source character set to the destination character set."}, {1397, "LabVIEW: (Hex 0x575) You have not wired a required input on this subVI."}, {1398, "LabVIEW: (Hex 0x576) The subVI cannot be inlined because there is a local variable in the block diagram."}, {1399, "LabVIEW: (Hex 0x577) The subVI cannot be inlined because a front panel terminal is not on the root diagram."}, {1400, "LabVIEW: (Hex 0x578) Attempted to read flattened data of a LabVIEW class. The flat data could not be converted to the requested type because the flat data is not the same as the requested type nor is it the same as any child class of the requested type."}, {1401, "LabVIEW: (Hex 0x579) Attempted to read flattened data of a LabVIEW class. The version of the class currently in memory is older than the version of the data. You must find a newer version of the class to load this data."}, {1402, "LabVIEW: (Hex 0x57A) Attempted to read flattened data of a LabVIEW class. The data was written by an old version of the class and the class in memory no longer supports loading and mutating data from that older version."}, {1403, "LabVIEW: (Hex 0x57B) Attempted to read flattened data of a LabVIEW class. The data is corrupt. LabVIEW could not interpret the data as any valid flattened LabVIEW class."}, {1404, "LabVIEW: (Hex 0x57C) Cannot insert or delete menu items while LabVIEW is tracking this menu. This error occurs when you use the Insert Menu Items or Delete Menu Items function to add or remove a menu item while a user is interacting with the menu."}, {1405, "LabVIEW: (Hex 0x57D) Operator Overloading info for a datatype has unsupported version number."}, {1406, "LabVIEW: (Hex 0x57E) Target file name to be searched is empty"}, {1407, "LabVIEW: (Hex 0x57F) Specified path to LV Targets Folder is not a Path"}, {1408, "LabVIEW: (Hex 0x580) Specified Target Folder path for the given LabVIEW Target is not valid"}, {1409, "LabVIEW: (Hex 0x581) Specified path for the given LabVIEW Target's directory is not a folder"}, {1410, "LabVIEW: (Hex 0x582) Specified LibDir in TargetDir chain has invalid path"}, {1411, "LabVIEW: (Hex 0x583) Specified LibDir in Target information file is not folder"}, {1412, "LabVIEW: (Hex 0x584) Specified path to Target's parent is not valid"}, {1413, "LabVIEW: (Hex 0x585) Specified path to Target's parent is not a folder"}, {1414, "LabVIEW: (Hex 0x586) Parent of a given target should not be contained within the target folder."}, {1415, "LabVIEW: (Hex 0x587) Given Target Class Name is already registered with different Target Path"}, {1416, "LabVIEW: (Hex 0x588) This Target Class Name is already registered with different device class"}, {1417, "LabVIEW: (Hex 0x589) This Target Class name has not been instantiated"}, {1418, "LabVIEW: (Hex 0x58A) Specified LabVIEW Target Name is empty"}, {1419, "LabVIEW: (Hex 0x58B) LabVIEW Target URL is empty"}, {1420, "LabVIEW: (Hex 0x58C) Application Instance Name or Target Alias is empty"}, {1421, "LabVIEW: (Hex 0x58D) Empty TargetClass name"}, {1422, "LabVIEW: (Hex 0x58E) Target is offline."}, {1423, "LabVIEW: (Hex 0x58F) Specified target syntax file for the given target could not be found"}, {1424, "LabVIEW: (Hex 0x590) Bad application reference."}, {1425, "LabVIEW: (Hex 0x591) Specified Application Instance not found"}, {1426, "LabVIEW: (Hex 0x592) Application Instance Name already in use under a given Target"}, {1427, "LabVIEW: (Hex 0x593) Application Instance of the given name exists but one or more properties do not match"}, {1428, "LabVIEW: (Hex 0x594) Application Instance has VIs running which need to be stopped and closed before executing the desired operations"}, {1429, "LabVIEW: (Hex 0x595) Command not supported by Target"}, {1430, "LabVIEW: (Hex 0x596) The path is empty or relative. You must use an absolute path."}, {1431, "LabVIEW: (Hex 0x597) This property cannot be used on a front panel with splitters."}, {1432, "LabVIEW: (Hex 0x598) The specified format cannot be used with floating point data. For example, hexadecimal notation is not a valid format for floating point numbers."}, {1433, "LabVIEW: (Hex 0x599) You cannot use absolute and relative time formats with complex numbers."}, {1434, "LabVIEW: (Hex 0x59A) The precision is greater than the maximum allowed value for this format."}, {1435, "LabVIEW: (Hex 0x59B) Values only from 0 to 8 are valid format values."}, {1436, "LabVIEW: (Hex 0x59C) Numeric precision cannot be negative."}, {1437, "LabVIEW: (Hex 0x59D) This application menu item has been removed. Menu item tags that existed in previous versions of LabVIEW as LabVIEW application item tags cannot be used."}, {1438, "LabVIEW: (Hex 0x59E) Archive version is later than the current LabVIEW version."}, {1439, "LabVIEW: (Hex 0x59F) A project library cannot be copied to the same folder as the original library because the new library files would conflict with the original library files on disk. You must specify a different location on disk when copying a project library."}, {1440, "LabVIEW: (Hex 0x5A0) The filename does not match the expected name."}, {1441, "LabVIEW: (Hex 0x5A1) An error has occurred in the build. Rebuild from the Project Explorer window to generate a more detailed error message."}, {1442, "LabVIEW: (Hex 0x5A2) The minimum pane size cannot be set to a value less than one."}, {1443, "LabVIEW: (Hex 0x5A3) Debug connection refused by specified server. Only one debug connection is allowed per application or shared library."}, {1444, "LabVIEW: (Hex 0x5A4) No VIs to download from application, connection closed."}, {1445, "LabVIEW: (Hex 0x5A5) Open VI Reference no longer matches VIs in memory by filename. A filename is no longer sufficient because the full name of a VI now includes any owning libraries."}, {1446, "LabVIEW: (Hex 0x5A6) The class of <b>object in</b> did not match the class of <b>target object</b> at run-time."}, {1447, "LabVIEW: (Hex 0x5A7) There was a name conflict while saving for previous. VIs in libraries are saved in the form LIBRARYNAME_VINAME. There is already a VI in this hierarchy with this name."}, {1448, "LabVIEW: (Hex 0x5A8) Bad type cast.  LabVIEW cannot treat the run-time value of this LabVIEW class as an instance of the given LabVIEW class."}, {1449, "LabVIEW: (Hex 0x5A9) Arrays must have at least one dimension and a maximum of 63 dimensions."}, {1450, "LabVIEW: (Hex 0x5AA) One or more untitled library dependencies exist. This file cannot be saved until all dependent files have been named."}, {1451, "LabVIEW: (Hex 0x5AB) One or more untitled dependencies exist. This file cannot be saved until all dependent files have been named."}, {1452, "LabVIEW: (Hex 0x5AC) This library was saved in an earlier version of LabVIEW. It must be loaded and saved in the current version of LabVIEW."}, {1453, "LabVIEW: (Hex 0x5AD) You may only set the vertical arrangement on a label, caption or free label."}, {1454, "LabVIEW: (Hex 0x5AE) LabVIEW classes cannot be flattened as XML in this version of LabVIEW."}, {1455, "LabVIEW: (Hex 0x5AF) Revert failed. This item has been edited in another context on this machine. Only that instance can be reverted."}, {1456, "LabVIEW: (Hex 0x5B0) Light cannot accept specified index."}, {1457, "LabVIEW: (Hex 0x5B1) Passed an invalid index to the clip plane."}, {1458, "LabVIEW: (Hex 0x5B2) Matrices must be arrays of 2 dimensions of size 4."}, {1459, "LabVIEW: (Hex 0x5B3) The scene contains a value that LabVIEW does not support."}, {1460, "LabVIEW: (Hex 0x5B4) Color component not in accepted range."}, {1461, "LabVIEW: (Hex 0x5B5) Bad value for the shininess of the material."}, {1462, "LabVIEW: (Hex 0x5B6) Cannot write this value.  This value is inherited from this node's parent."}, {1463, "LabVIEW: (Hex 0x5B7) This scene is missing expected nodes or contains nodes that LabVIEW does not support."}, {1464, "LabVIEW: (Hex 0x5B8) Fog start and fog end cannot be the same."}, {1465, "LabVIEW: (Hex 0x5B9) Bad value for point size. You must pass a positive number for this value."}, {1466, "LabVIEW: (Hex 0x5BA) Bad value. You must pass a positive number for this value."}, {1467, "LabVIEW: (Hex 0x5BB) Bad value. Value must be 0 < Value <= 1."}, {1468, "LabVIEW: (Hex 0x5BC) Specified ability not supported by the library."}, {1469, "LabVIEW: (Hex 0x5BD) Specified ability already exists."}, {1470, "LabVIEW: (Hex 0x5BE) Specified folder is outside the library."}, {1471, "LabVIEW: (Hex 0x5BF) Bad value passed for spotlight cutoff."}, {1472, "LabVIEW: (Hex 0x5C0) Bad value passed for the exponent of a spotlight."}, {1473, "LabVIEW: (Hex 0x5C1) Bad value passed for light attenuation."}, {1474, "LabVIEW: (Hex 0x5C2) Bad value or array configuration."}, {1475, "LabVIEW: (Hex 0x5C3) Bad pixmap cluster."}, {1476, "LabVIEW: (Hex 0x5C4) Cannot add the specified node."}, {1477, "LabVIEW: (Hex 0x5C5) An index in the mesh is greater than the number of elements in the element array."}, {1478, "LabVIEW: (Hex 0x5C6) Bad texture index size."}, {1479, "LabVIEW: (Hex 0x5C7) Access denied. The language configured on this target is incompatible with the host LabVIEW language."}, {1480, "LabVIEW: (Hex 0x5C8) LabVIEW did not generate documentation files because some of the files are read-only."}, {1481, "LabVIEW: (Hex 0x5C9) The libraries that support 3D rendering and operations are missing. This property or method cannot function without these libraries."}, {1482, "LabVIEW: (Hex 0x5CA) The view direction either cannot be determined or is colinear with the up vector."}, {1483, "LabVIEW: (Hex 0x5CB) Cannot change width of the plot legend when you configure the plot legend to automatically resize, or if the legend has more than one entry and you arrange the plot legend horizontally."}, {1484, "LabVIEW: (Hex 0x5CC) LabVIEW cannot inline the subVI into its calling VIs because the block diagram of the subVI contains an implicit control reference."}, {1485, "LabVIEW: (Hex 0x5CD) LabVIEW cannot inline the subVI into its calling VIs because the block diagram of the subVI contains an implicit Property Node or Invoke Node."}, {1486, "LabVIEW: (Hex 0x5CE) This property or method cannot be executed on a reference that refers to a LabVIEW class loaded in a different application instance."}, {1487, "LabVIEW: (Hex 0x5CF) This control cannot be sized."}, {1488, "LabVIEW: (Hex 0x5D0) The migration file cannot load because it is no longer supported."}, {1489, "LabVIEW: (Hex 0x5D1) The migration file cannot load because its content is not valid or is corrupt."}, {1490, "LabVIEW: (Hex 0x5D2) The migration file cannot load because it makes references to data that does not exist or is invalid."}, {1491, "LabVIEW: (Hex 0x5D3) If you obtain a queue reference in one application instance, you cannot use that queue reference in another application instance."}, {1492, "LabVIEW: (Hex 0x5D4) If you obtain a notifier reference in one application instance, you cannot use that notifier reference in another application instance."}, {1493, "LabVIEW: (Hex 0x5D5) The save operation failed because multiple files of the same name cannot be saved into a single LLB. To correct this error, save to a folder instead of an LLB."}, {1494, "LabVIEW: (Hex 0x5D6) Textures are limited to dimensions of 512 X 512."}, {1495, "LabVIEW: (Hex 0x5D7) Meshes cannot share empty arrays."}, {1496, "LabVIEW: (Hex 0x5D8) There must be enough data in the array for the given color or normal binding mode."}, {1497, "LabVIEW: (Hex 0x5D9) Cannot unlock a library for edit when instances in running VIs exist."}, {1498, "LabVIEW: (Hex 0x5DA) Library has errors. Fix the errors before attempting this operation."}, {1499, "LabVIEW: (Hex 0x5DB) Library has edits in another context. Sync up changes before attempting this operation."}, {1500, "LabVIEW: (Hex 0x5DC) If you obtain a user event reference in one application instance, you cannot use that user event reference in another
